vi "get_last_value.vi"(8 "error in (no error)":errorcluster, 11 "MeasurementDatalvclass in":refnum<class "MeasurementDatalvclass.lvclass">) -> (0 "error out":errorcluster, 2 "output":u16[](array[numeric]), 3 "MeasurementDatalvclass out":refnum<class "MeasurementDatalvclass.lvclass">)   [LabVIEW 2017, in "MeasurementDatalvclass.lvclass"]
doc: "Get the last value of measurement data"
uses:
  MeasurementDatalvclass.lvclass
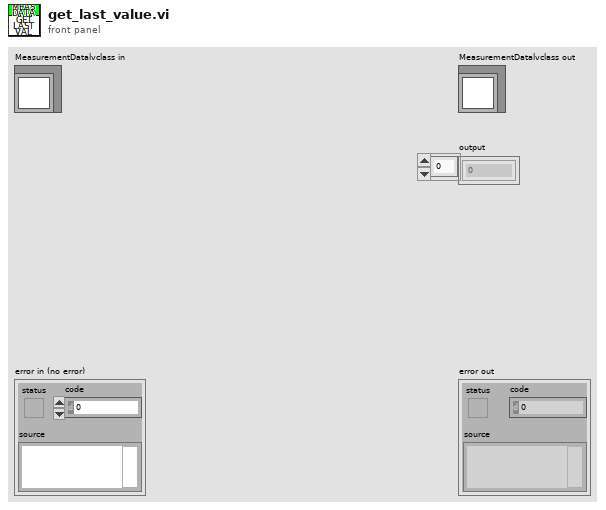
[diagram p1: front panel]
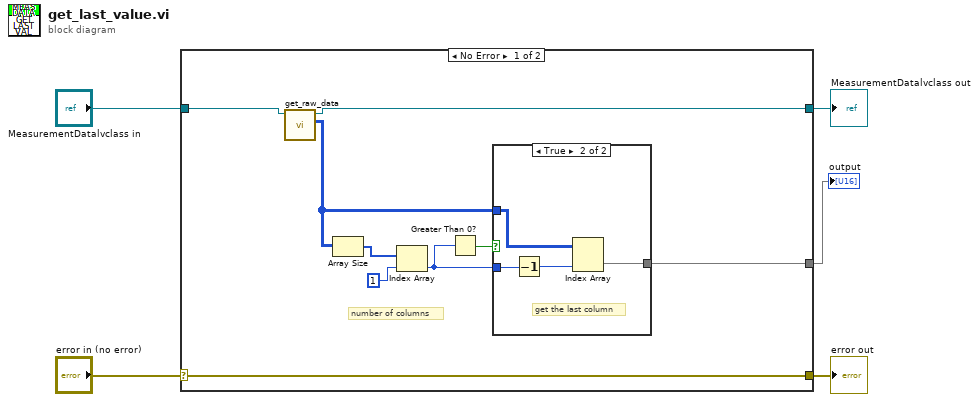
[diagram p0: block diagram]
diagram:
  n1 = case shown="No Error" "error in (no error)" {
    selector: "error in (no error)" -> [w14 w20]
    tunnel: [w14 w20] -> w4
    tunnel: [w12 w19] -> w2
    tunnel: "MeasurementDatalvclass in" -> [w13 w19]
    tunnel: [w6 _] -> w1
    frame No Error {
      # "number of columns"
      n2 = call-dynamic "get_raw_data.vi"("MeasurementResult in"=w13) -> ("raw_data"=w7:u16[][], "MeasurementResult out"=w12:refnum<class "MeasurementDatalvclass.lvclass">)  [unwired: 8 in, 1 out]
      n3 = Array Size(array=w7) -> (size(s)=w11:i32[])
      n4 = Index Array(array=w11, index=1) -> (element=w8:i32)
      n5 = Greater Than 0?(x=w8) -> (x > 0?=w9:bool)
      n6 = case shown="True" w9 {
        tunnel: w8 -> [_ w18]
        tunnel: w7 -> [_ w16]
        tunnel: [_ w15] -> w6
        frame False {
        }
        frame True {
          # "get the last column"
          n7 = Decrement(x=w18) -> (x-1=w17:i32)
          n8 = Index Array(array=w16, index (col)=w17) -> (element=w15:u16[])  [unwired: 1 in]
        }
      }
    }
    frame Error {
    }
  }
  "error out" <- w4
  "MeasurementDatalvclass out" <- w2
  "output" <- w1
